vi "Snap.vi"(8 "error in (no error)":errorcluster, 11 "reference in":refnum<class "Camera_Sim.lvclass">) -> (0 "error out":errorcluster, 2 "Image Out":T1, 3 "reference out":refnum<class "Camera_Sim.lvclass">)   [LabVIEW 2017, in "Camera_Sim.lvclass"]
doc: "Snaps a single image. Does not require Start and Stop Acquisition."
uses:
  Camera_Sim.lvclass
  <vilib>/vision/Image Controls.llb/IMAQ Image.ctl
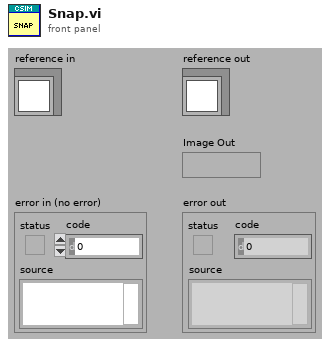
[diagram p1: front panel]
types:
  T1 = typedef "IMAQ Image.ctl" = refnum<image>
  T2 = typedef "CameraSim.lvclass/ObjectAttributes.ctl" = cluster{"Connected":bool, "Image Out":T1, "Frame Number":u32, "Path":path}
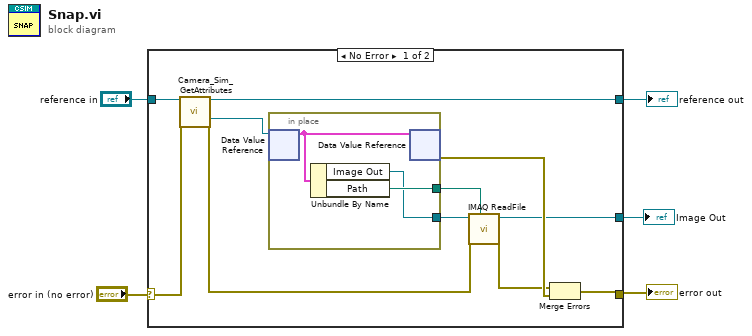
[diagram p0: block diagram]
diagram:
  n1 = case shown="No Error" "error in (no error)" {
    selector: "error in (no error)" -> [w15 w21]
    tunnel: [w13 w21] -> w4
    tunnel: [w12 w20] -> w2
    tunnel: "reference in" -> [w16 w20]
    tunnel: [w6 _] -> w1
    frame No Error {
      n2 = call "Camera_Sim_GetAttributes.vi"("reference in"=w16, "error in (no error)"=w15) -> ("reference out"=w12:refnum<class "Camera_Sim.lvclass">, "DataRef"=w11:refnum<data-value>, "error out"=w9:errorcluster)  [unwired: 10 in, 1 out]
      n3 = in-place {
        in-place-border: [w18] -> w10
        in-place-border: [w17] -> w8
        n4 = in-place-dvr #1(w11) -> (w19:T2)  [unwired: 1 out]
        n5 = Unbundle By Name(w19) -> ("Image Out"=w17:T1, "Path"=w18:path)
        n6 = in-place-dvr #1(w19) -> (w14:errorcluster)  [unwired: 1 out]
      }
      n7 = call "IMAQ ReadFile"("File Path"=w10, "error in (no error)"=w9, "Image"=w8) -> ("error out"=w7:errorcluster, "Image Out"=w6:T1)  [unwired: 2 in, 5 out]
      n8 = Merge Errors(w7, w14) -> (w13:errorcluster)
    }
    frame Error {
    }
  }
  "error out" <- w4
  "reference out" <- w2
  "Image Out" <- w1
